vi "Read Axis Cfg.vi"(8 "error in (no error)":errorcluster, 11 "Axis in":refnum<class "Axis.lvclass">) -> (0 "error out":errorcluster, 3 "Axis out":refnum<class "Axis.lvclass">)   [LabVIEW 2018, in "Axis.lvlib" / "Axis.lvclass"]
uses:
  Axis.lvclass
  Axis.lvclass/Axis.ctl
  PPLs/Configuration/Configuration.lvlibp/Configuration.lvclass
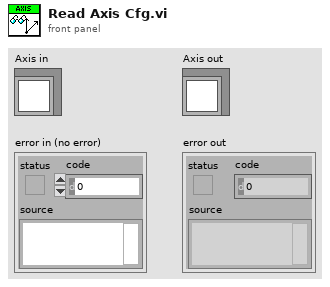
[diagram p1: front panel]
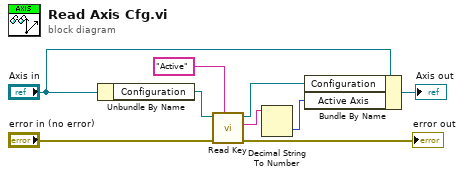
[diagram p0: block diagram]
diagram:
  n1 = Unbundle By Name("Axis in") -> ("Configuration"=w7:refnum<class "Configuration.lvclass">)
  n2 = call "Read Key.vi"("Key:"="Active", "error in"="error in (no error)", "Configuration in"=w7) -> ("error out"=→"error out":errorcluster, "Value"=w3:string, "Configuration out"=w6:refnum<class "Configuration.lvclass">)  [unwired: 6 in]
  n3 = Decimal String To Number(string=w3) -> (number=w2:i32)  [unwired: 2 in, 1 out]
  n4 = Bundle By Name(cluster="Axis in", "Configuration"=w6, "Active Axis"=w2) -> (→"Axis out":refnum<class "Axis.lvclass">)
